vi "Max Panels.vi"(8 "error in (no error)":errorcluster, 11 "SubPanel 3x3 View in":refnum<class "SubPanel 3x3 View.lvclass">) -> (0 "error out":errorcluster, 1 "Max Panels":i32, 3 "SubPanel 3x3 View out":refnum<class "SubPanel 3x3 View.lvclass">)   [LabVIEW 2012, in "Win8uiDemo.lvlib" / "SubPanel 3x3 View.lvclass"]
uses:
  SubPanel 3x3 View.lvclass
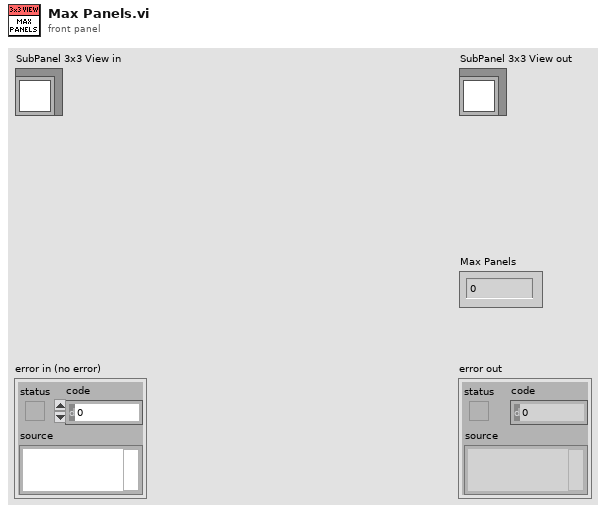
[diagram p1: front panel]
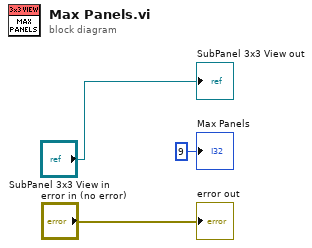
[diagram p0: block diagram]
diagram:
  "error out" <- "error in (no error)"
  "SubPanel 3x3 View out" <- "SubPanel 3x3 View in"
  "Max Panels" <- 9 ("Max Panels")
